vi "SpectralEmbedding.vi"(8 "error in":errorcluster) -> (0 "error out":errorcluster, 3 "out":refnum<class "SpectralEmbedding.lvclass">)   [LabVIEW 2020]
doc: "Spectral embedding for non-linear dimensionality reduction.\n\n Forms an affinity matrix given by the specified function and\n applies spectral decomposition to the corresponding graph laplacian.\n The resulting transformation is given by the value of the\n eigenvectors for each data point.\n\n Note : Laplacian Eigenmaps is the actual algorithm implemented here.\n\n Read more in the :ref:`User Guide <spectral_embedding>`.\n\n Parameters\n ----------\n n_components : int, default=2\n The dimension of the projected subspace.\n\n affinity : {'nearest_neighbors', 'rbf', 'precomputed', 'precomputed_nearest_neighbors'} or callable, default='nearest_neighbors'\n How to construct the affinity matrix.\n - 'nearest_neighbors' : construct the affinity matrix by computing a\n graph of nearest neighbors.\n - 'rbf' : construct the affinity matrix by computing a radial basis\n function (RBF) kernel.\n - 'precomputed' : interpret ``X`` as a precomputed affinity matrix.\n - 'precomputed_nearest_neighbors' : interpret ``X`` as a sparse graph\n of precomputed nearest neighbors, and constructs the affinity matrix\n by selecting the ``n_neighbors`` nearest neighbors.\n - callable : use passed in function as affinity\n the function takes in data matrix (n_samples, n_features)\n and return affinity matrix (n_samples, n_samples).\n\n gamma : float, default=None\n Kernel coefficient for rbf kernel. If None, gamma will be set to\n 1/n_features.\n\n random_state : int, RandomState instance or None, default=None\n Determines the random number generator used for the initialization of\n the lobpcg eigenvectors when ``solver`` == 'amg'. Pass an int for\n reproducible results across multiple function calls.\n See :term: `Glossary <random_state>`.\n\n eigen_solver : {'arpack', 'lobpcg', 'amg'}, default=None\n The eigenvalue decomposition strategy to use. AMG requires pyamg\n to be installed. It can be faster on very large, sparse problems.\n If None, then ``'arpack'`` is used.\n\n n_neighbors : int, default=None\n Number of nearest neighbors for nearest_neighbors graph building.\n If None, n_neighbors will be set to max(n_samples/10, 1).\n\n n_jobs : int, default=None\n The number of parallel jobs to run.\n ``None`` means 1 unless in a :obj:`joblib.parallel_backend` context.\n ``-1`` means using all processors. See :term:`Glossary <n_jobs>`\n for more details.\n\n Attributes\n ----------\n embedding_ : ndarray of shape (n_samples, n_components)\n Spectral embedding of the training matrix.\n\n affinity_matrix_ : ndarray of shape (n_samples, n_samples)\n Affinity_matrix constructed from samples or precomputed.\n\n n_neighbors_ : int\n Number of nearest neighbors effectively used.\n\n \nAvailable methods:\nFit\nFit Transform\nGet Attributes\nGet Params\nSet Params"
uses:
  SpectralEmbedding.lvclass
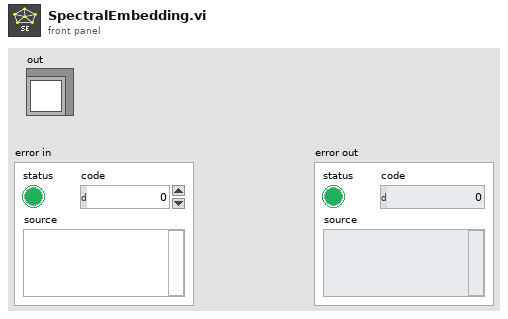
[diagram p1: front panel]
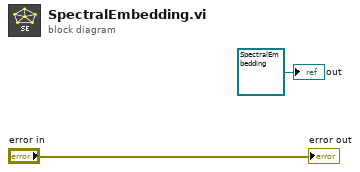
[diagram p0: block diagram]
diagram:
  "out" <- refnum<class "SpectralEmbedding.lvclass"> refnum ("model")
  "error out" <- "error in"
